vi "priorCoord (SubVI).vi"(10 "startCoord":cluster{"x start":i32, "y start":i32}, 11 "paneCoord":cluster{"x abs ":i32, "y abs":i32}) -> (3 "relatCoord":cluster{"x relat ":i32, "y relat":i32})   [LabVIEW 2011]
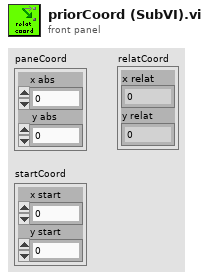
[diagram p1: front panel]
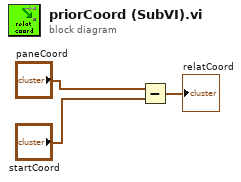
[diagram p0: block diagram]
diagram:
  n1 = Subtract(x="paneCoord", y="startCoord") -> (x-y=→"relatCoord":cluster{i32, i32})
